vi "Select Channels and Update Properties.vi"(7 "Generate?":bool, 8 "error in (no error)":errorcluster, 11 "Node Ptr":u64) -> (0 "error out":errorcluster)   [LabVIEW 2021, in "LIN Frame Protection Addon System Explorer.lvlib"]
uses:
  LIN Frame Protection Addon System Explorer.lvlib
  Shared/LIN Frame Protection Addon Shared.lvlib
  <vilib>/NI VeriStand/Custom Device Tools/Custom Device Utility Library/Custom Device Utility Library.lvlib
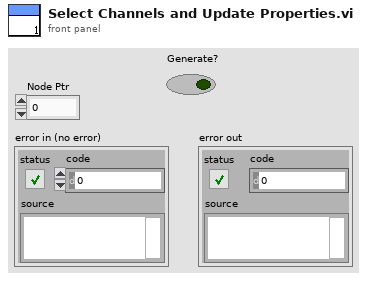
[diagram p1: front panel]
types:
  T1 = typedef "LIN Frame Protection Addon Shared.lvlib/FrameConfiguration.ctl" = cluster{"Input Channels":T2[], "Schedule_SumOfDelays":cluster{"Index":i32, "Delays":dbl[]}, "Rolling Counter Count":dbl, "PCL Count":u64, "Max Count":dbl, "Frame ID":u32, "Rolling Counter":T2, "CRC":T2, "Frame Name":string, "Cluster":string, "Database":string, "Protection Type":T3}
  T2 = typedef "LIN Frame Protection Addon Shared.lvlib/InputChannelConfiguration.ctl" = cluster{"Start Bit":i32, "Name":string, "Node Path":string, "Number of bits":i32, "Scale":dbl, "Offset":dbl, "Data Type":u32}
  T3 = typedef "LIN Frame Protection Addon Shared.lvlib/Protection Type.ctl" = enum16{"Checksum", "CRC", "None (Counter Only)"}
  T4 = typedef "Custom Device API.lvlib/Custom Device Item Ref.ctl" = u64
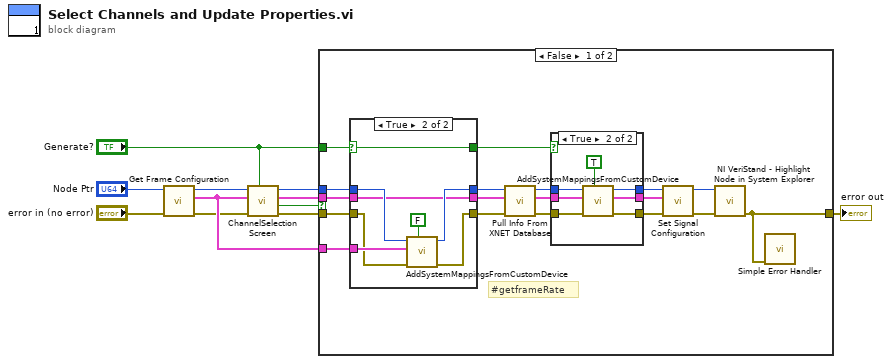
[diagram p0: block diagram]
diagram:
  n1 = call "Get Frame Configuration.vi"("error in"="error in (no error)", "Parent Ref"="Node Ptr") -> ("error out"=w4:errorcluster, "Selected Channels"=w10:T1, "Parent Ref Out"=w3:T4)  [unwired: 7 in]
  n2 = call "ChannelSelectionScreen.vi"("Generate?"="Generate?", "error in"=w4, "Frame Configuration"=w10, "Parent Ref"=w3) -> ("error out"=w5:errorcluster, "Cancelled?"=w7:bool, "Frame Configuration out"=w11:T1, "Parent Ref Out"=w6:T4)  [unwired: 4 in]
  n3 = case shown="False" w7 {
    tunnel: w5 -> [w21 w52]
    tunnel: w6 -> [w23 _]
    tunnel: w11 -> [w14 _]
    tunnel: [w16 w52] -> w9
    tunnel: w10 -> [w19 _]
    tunnel: "Generate?" -> [w13 _]
    frame False {
      # "#getframeRate"
      n4 = case shown="True" w13 {
        selector: w13 -> [w30 w34]
        tunnel: w23 -> [w31 w41]
        tunnel: [w31 w40] -> w22
        tunnel: w21 -> [w32 w37]
        tunnel: [w32 w36] -> w20
        tunnel: w19 -> [_ w38]
        tunnel: [w33 w35] -> w15
        tunnel: w14 -> [w33 w35]
        tunnel: [w30 w34] -> w12
        frame False {
        }
        frame True {
          n5 = call "AddSystemMappingsFromCustomDevice.vi"("Add? (T)"=FALSE, "error in"=w37, "Frame Configuration"=w38, "Node Ptr"=w41) -> ("error out"=w36:errorcluster, "Section Ref out"=w40:T4)  [unwired: 5 in, 1 out]
        }
      }
      n6 = call "Pull Info From XNET Database.vi"("error in"=w20, "Frame Configuration"=w15, "Parent Ref"=w22) -> ("error out"=w27:errorcluster, "Frame Configuration"=w18:T1, "Item Ref out"=w25:T4)  [unwired: 6 in]
      n7 = case shown="True" w12 {
        tunnel: w27 -> [w42 w51]
        tunnel: [w42 w50] -> w26
        tunnel: w25 -> [w44 w49]
        tunnel: [w44 w48] -> w24
        tunnel: w18 -> [w43 w46]
        tunnel: [w43 w45] -> w17
        frame False {
        }
        frame True {
          n8 = call "AddSystemMappingsFromCustomDevice.vi"("Add? (T)"=TRUE, "error in"=w51, "Frame Configuration"=w46, "Node Ptr"=w49) -> ("error out"=w50:errorcluster, "Frame Configuration out"=w45:T1, "Section Ref out"=w48:T4)  [unwired: 5 in]
        }
      }
      n9 = call "Set Signal Configuration.vi"("error in"=w26, "Selected Channels"=w17, "Parent Ref"=w24) -> ("error out"=w28:errorcluster, "Parent Ref Out"=w29:T4)  [unwired: 7 in]
      n10 = call <vilib>:"NI VeriStand - Highlight Node in System Explorer.vi"("error in (no error)"=w28, "Item Ref in"=w29) -> ("error out"=w16:errorcluster)  [unwired: 8 in, 1 out]
      n11 = call <vilib>:"Simple Error Handler.vi"("error in (no error)"=w16) -> ()  [unwired: 4 in, 5 out]
    }
    frame True {
    }
  }
  "error out" <- w9
